vi "Change AO Gain On Fly or Not (scaled data).vi"() -> ()   [LabVIEW 2015]
doc: "I. Description:\nThis example demonstrates how to output a continuous periodic waveform using an internal sample clock.\n\nII. Instructions for Running:\n1. Select the Physical Channel to correspond to where your signal is output on the DAQ device.\n2. Enter the Minimum and Maximum Voltage Ranges\n3. Specify the Desired Frequency of the output Waveform\n4. Enter the Waveform Information. See the documentation of the Waveform Buffer Generation SubVI for information on each parameter.\n\nIII. Block Diagram Steps:\n1. Create an Analog Output Voltage channel.\n2. Call the DAQmx Timing (Use Waveform) VI which sets the sample clock rate based on the input waveform parameters, and set the sample mode to Continuous.\n3. Write the waveform to the output buffer.\n4. Call the Start VI.\n5. Loop continuously until the user presses the Stop button. Check for errors every 100 ms using the Is Task Done? VI\n6. Clear the Task\n7. Use the popup dialog box to display an error or warning if any.\n\nIV. I/O Connections Overview:\nMake sure your signal output terminal matches the Physical Channel I/O Control. For further connection information, refer to your hardware reference manual."
uses:
  <vilib>/DAQmx/create/channels.llb/DAQmx Create Channel (AO-Voltage-Basic).vi
  <vilib>/Utility/error.llb/DialogType.ctl
  <vilib>/DAQmx/configure/timing.llb/DAQmx Timing (Sample Clock).vi
  <vilib>/DAQmx/write.llb/DAQmx Write (Analog 2D DBL NChan NSamp).vi
  <resource>/objmgr/daqmx.rc
panel:
  in  "AO Idle State":bool=TRUE
  in  "Gain Setting 2":u16(ring) items=["0 dB Gain"=0, "20 dB Gain"=2, "40 dB Gain"=4]
  in  "AO Channel 2":u16(ring)=1536 items=["AO 0"=1536, "AO 1"=1540]
  in  "AO Channel":u16(ring)=1536 items=["AO 0"=1536, "AO 1"=1540]
  in  "Gain Setting":u16(ring) items=["0 dB Gain"=0, "20 dB Gain"=2, "40 dB Gain"=4]
  out "Resulting Frequency":dbl=1000.0000002037268 format="%.2f"
  in  "Cycles per Buffer":i32=5
  in  "Waveform Type":T1(ring)
  in  "Desired Frequency":dbl=1000.0 format="%.2f"
  in  "Samples per Buffer":dbl=250.0
  in  "Amplitude":dbl=10.0 format="%0.2p"
  out "Waveform Graph":dbl[](graph)=[0.0, 1.2533323356430426, 2.486898871648548, 3.6812455268467796, 4.817536741017153, 5.877852522924731, 6.845471059286887, 7.705132427757892, 8.443279255020151, 9.048270524660195, 9.510565162951536, 9.822872507286887, 9.980267284282716, 9.980267284282716, 9.822872507286887, 9.510565162951536, 9.048270524660195, 8.443279255020151, 7.705132427757892, 6.845471059286886, 5.877852522924731, 4.817536741017152, 3.681245526846779, 2.4868988716485467, 1.2533323356430417, -1.7390602846667491e-15, -1.2533323356430437, -2.4868988716485503, -3.6812455268467814, -4.817536741017156, -5.877852522924734, -6.84547105928689, -7.705132427757895, -8.443279255020155, -9.048270524660198, -9.51056516295154, -9.82287250728689, -9.98026728428272, -9.980267284282718, -9.82287250728689, -9.510565162951536, -9.048270524660198, -8.443279255020151, -7.705132427757895, -6.845471059286886, -5.877852522924733, -4.817536741017151, -3.6812455268467796, -2.4868988716485454, -1.2533323356430413, 3.432800918523604e-15, 1.253332335643045, 2.486898871648552, 3.6812455268467836, 4.8175367410171575, 5.877852522924736, 6.845471059286892, 7.705132427757898, 8.443279255020155, 9.048270524660202, 9.51056516295154, 9.822872507286894, 9.98026728428272, 9.980267284282721, 9.82287250728689, 9.51056516295154, 9.048270524660197, 8.443279255020153, 7.705132427757892, 6.845471059286887, 5.877852522924729, 4.817536741017152, 3.681245526846776, 2.486898871648546, 1.2533323356430375, -3.4618575367462157e-15, -1.2533323356430486, -2.486898871648553, -3.6812455268467863, -4.817536741017159, -5.877852522924738, -6.8454710592868935, -7.705132427757898, -8.443279255020158, -9.0482705246602, -9.510565162951544, -9.82287250728689, -9.980267284282723, -9.980267284282718, -9.822872507286894, -9.510565162951536, -9.0482705246602, -8.44327925502015, -7.705132427757895, -6.845471059286884, -5.877852522924731, -4.817536741017148, -3.6812455268467765, -2.486898871648541, -1.253332335643037, 8.040009630283507e-15, 1.2533323356430497, 2.4868988716485565, 3.681245526846788, 4.817536741017162, 5.877852522924741, 6.845471059286895, 7.705132427757902, 8.443279255020158, 9.048270524660204, 9.510565162951542, 9.822872507286894, 9.98026728428272, 9.980267284282721, 9.822872507286888, 9.51056516295154, 9.048270524660195, 8.443279255020153, 7.705132427757889, 6.845471059286886, 5.8778525229247265, 4.8175367410171495, 3.681245526846773, 2.486898871648542, 1.2533323356430341, -8.543513119185775e-15, -1.2533323356430521, -2.4868988716485583, -3.6812455268467903, -4.817536741017165, -5.8778525229247425, -6.8454710592869, -7.705132427757903, -8.443279255020164, -9.048270524660204, -9.510565162951547, -9.822872507286894, -9.980267284282725, -9.98026728428272, -9.822872507286894, -9.510565162951538, -9.048270524660198, -8.443279255020151, -7.705132427757892, -6.845471059286885, -5.877852522924727, -4.817536741017148, -3.6812455268467725, -2.4868988716485405, -1.2533323356430324, 8.901516676540489e-15, 1.253332335643055, 2.486898871648558, 3.681245526846794, 4.817536741017164, 5.877852522924746, 6.845471059286898, 7.705132427757906, 8.44327925502016, 9.048270524660207, 9.510565162951544, 9.822872507286897, 9.980267284282721, 9.980267284282723, 9.82287250728689, 9.51056516295154, 9.048270524660195, 8.443279255020151, 7.705132427757889, 6.845471059286884, 5.877852522924726, 4.817536741017146, 3.681245526846771, 2.486898871648538, 1.2533323356430321, -1.2734388196711244e-14, -1.253332335643054, -2.4868988716485623, -3.681245526846791, -4.817536741017168, -5.8778525229247425, -6.8454710592869015, -7.705132427757903, -8.443279255020164, -9.048270524660204, -9.510565162951547, -9.822872507286894, -9.980267284282725, -9.98026728428272, -9.822872507286892, -9.510565162951536, -9.048270524660197, -8.44327925502015, -7.705132427757889, -6.845471059286883, -5.877852522924725, -4.817536741017146, -3.6812455268467694, -2.4868988716485387, -1.253332335643029, 1.1011590944631777e-14, 1.2533323356430581, 2.4868988716485605, 3.6812455268467965, 4.8175367410171654, 5.877852522924749, 6.845471059286899, 7.705132427757909, 8.443279255020162, 9.04827052466021, 9.510565162951545, 9.822872507286899, 9.980267284282723, 9.980267284282725, 9.82287250728689, 9.51056516295154, 9.048270524660195, 8.443279255020151, 7.7051324277578885, 6.845471059286883, 5.877852522924724, 4.817536741017144, 3.681245526846769, 2.486898871648535, 1.253332335643029, -1.612208630485945e-14, -1.2533323356430577, -2.4868988716485663, -3.6812455268467956, -4.8175367410171726, -5.877852522924747, -6.845471059286907, -7.705132427757906, -8.443279255020169, -9.048270524660207, -9.510565162951552, -9.822872507286895, -9.980267284282728, -9.980267284282721, -9.822872507286895, -9.510565162951538, -9.048270524660198, -8.44327925502015, -7.70513242775789, -6.845471059286881, -5.877852522924724, -4.817536741017143, -3.681245526846767, -2.486898871648535, -1.2533323356430262] caption="Output Waveform"
  in  "Physical Channels":tag="PXI1Slot2/ao0:1"
  in  "Minimum Value":dbl=-10.0 format="%0.2f"
  in  "Maximum Value":dbl=10.0 format="%0.2f"
  in  "stop":bool
  # "For instructions, select Help>>Show Context Help"
  # "Channel Parameters"
  # "Timing Parameters"
  # "Waveform Information"
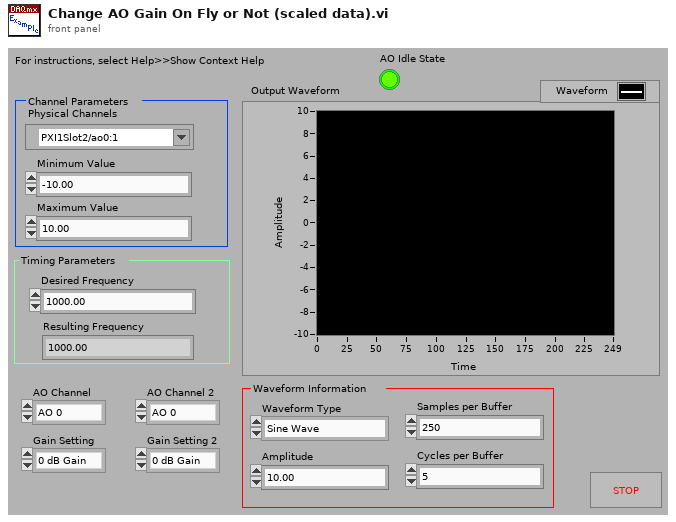
[diagram p1: front panel]
types:
  T1 = enum16{"Sine Wave", "Triangle Wave", "Square Wave", "Sawtooth Wave"}
  T2 = typedef "DialogType.ctl" = u16
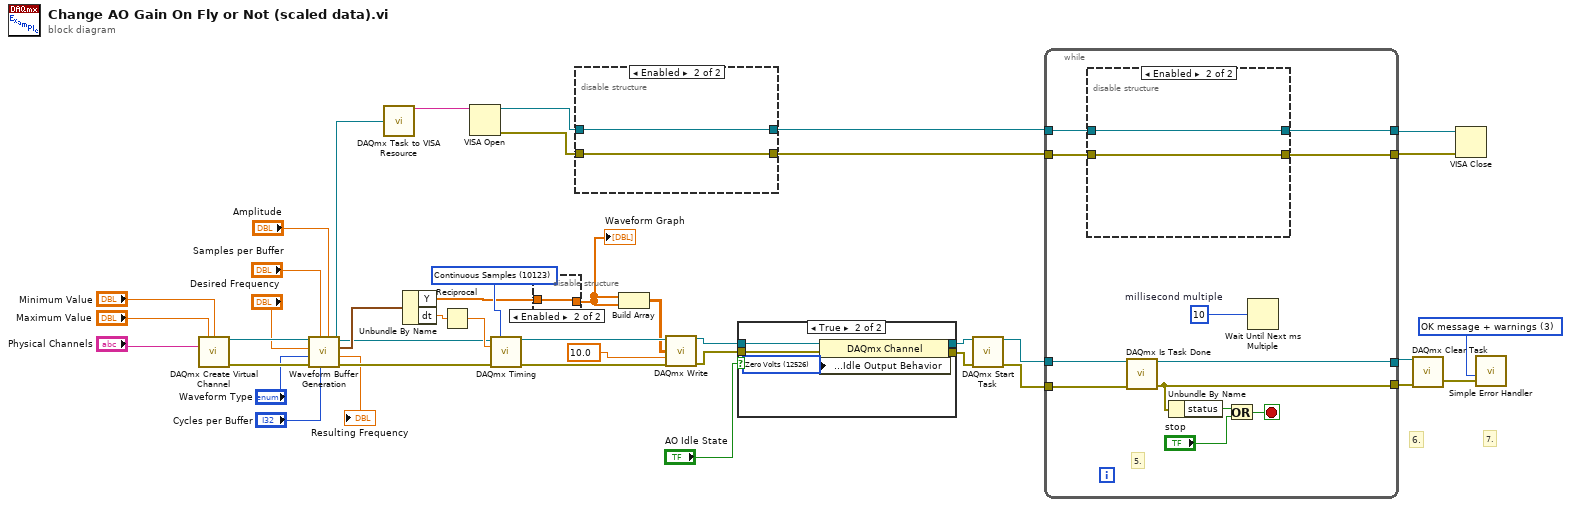
[diagram p0: block diagram]
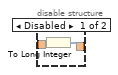
[diagram p3: hidden frame]
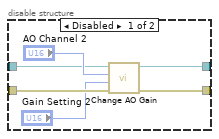
[diagram p4: hidden frame]
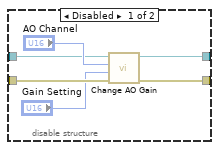
[diagram p5: hidden frame]
diagram:
  w15 = 10123 items=["Finite Samples"=10178, "Continuous Samples"=10123, "Hardware Timed Single Point"=12522] ("sample mode")
  w32 = T2 3 items=["no dialog", "OK message", "continue or stop message", "OK message + warnings", "continue/stop + warnings"] ("type of dialog (OK msg:1)")
  # "7."
  # "6."
  n1 = call-poly <vilib>:"DAQmx Create Virtual Channel.vi"("maximum value"="Maximum Value", "minimum value"="Minimum Value", "physical channels"="Physical Channels") -> ("task out"=w28:refnum<k21>, "error out"=w27:errorcluster)  [unwired: 11 in]
  n2 = call "Waveform Buffer Generation.vi"("Amplitude"="Amplitude", "Cycles per Buffer"="Cycles per Buffer", "Samples per Buffer"="Samples per Buffer", "error in (no error)"=w27, "Waveform Type"="Waveform Type", "Desired Frequency"="Desired Frequency", "task/channels in"=w28) -> ("error out"=w29:errorcluster, "Resulting Frequency"=→"Resulting Frequency":dbl, "Waveform"=w18:waveform(dbl), "task out"=w10:refnum<k21>)  [unwired: 1 out]
  n3 = call "DAQmx Task to VISA Resource.vi"("task out"=w10) -> ("VISAName"=w21:string)
  n4 = Unbundle By Name(w18) -> ("Y"=w11:dbl[], "dt"=w17:dbl)
  n5 = Reciprocal(x=w17) -> (1/x=w16:dbl)
  n6 = VISA Open(VISA resource name=w21) -> (VISA resource name=w7:refnum<visa-resource-name>, error out=w6:errorcluster)  [unwired: 4 in]
  n7 = call-poly <vilib>:"DAQmx Timing.vi"("task/channels in"=w10, "sample mode"=w15, "rate"=w16, "error in"=w29) -> ("task out"=w35:refnum<k21>, "error out"=w34:errorcluster)  [unwired: 10 in]
  n8 = disable-structure shown="Enabled" {
    disable-tunnel: [w43 w44] -> w12
    disable-tunnel: w11 -> [w42 w44]
    frame Disabled {
      n9 = To Long Integer(number=w42) -> (32bit integer=w43:i32[])
    }
    frame Enabled {
    }
  }
  "Waveform Graph" <- w12
  n10 = disable-structure shown="Enabled" {
    disable-tunnel: w6 -> [w50 w51]
    disable-tunnel: [w49 w52] -> w9
    disable-tunnel: [w48 w51] -> w8
    disable-tunnel: w7 -> [w45 w52]
    frame Disabled {
      n11 = call "Change AO Gain.vi"("error in"=w50, "Gain Setting"="Gain Setting 2", "AO Channel"="AO Channel 2", "VISA resource name 2"=w45) -> ("error out"=w48:errorcluster, "VISA resource name"=w49:refnum<visa-resource-name>)  [unwired: 4 in]
    }
    frame Enabled {
    }
  }
  n12 = Build Array(w12, w12) -> (w14:dbl[][])
  n13 = call-poly <vilib>:"DAQmx Write.vi"("task/channels in"=w35, "data"=w14, "timeout"=10.0 ("Wirite Timeout"), "error in"=w34) -> ("task out"=w4:refnum<k21>, "error out"=w3:errorcluster)  [unwired: 9 in, 1 out]
  n14 = case shown="True" "AO Idle State" {
    tunnel: w4 -> [w54 w58]
    tunnel: w3 -> [w53 w57]
    tunnel: [w54 w56] -> w2
    tunnel: [w53 w55] -> w1
    frame False {
    }
    frame True {
      w59 = 12526 items=["Zero Volts"=12526, "High Impedance"=12527, "Maintain Existing Value"=12528] ("AO.IdleOutputBehavior")
      n15 = property class="DAQmx Channel"(reference=w58, error in=w57, "Analog Output:General Properties:Output Configuration:Idle Output Behavior"=w59) -> (reference out=w56:refnum<k21>, error out=w55:errorcluster)
    }
  }
  n16 = call <vilib>:"DAQmx Start Task.vi"("task/channels in"=w2, "error in"=w1) -> ("task out"=w33:refnum<k21>, "error out"=w37:errorcluster)  [unwired: 12 in]
  n17 = while {
    tunnel: w33 -> [w71]
    tunnel: [w70] -> w31
    tunnel: w37 -> [w69]
    tunnel: [w68] -> w30
    tunnel: w9 -> [w60]
    tunnel: w8 -> [w63]
    tunnel: [w62] -> w20
    tunnel: [w61] -> w19
    stop <- w66 stop-if-true
    w67 = u32 10  # millisecond multiple
    # "5."
    n18 = disable-structure shown="Enabled" {
      disable-tunnel: w63 -> [w77 w78]
      disable-tunnel: [w76 w79] -> w62
      disable-tunnel: [w75 w78] -> w61
      disable-tunnel: w60 -> [w72 w79]
      frame Disabled {
        n19 = call "Change AO Gain.vi"("error in"=w77, "Gain Setting"="Gain Setting", "AO Channel"="AO Channel", "VISA resource name 2"=w72) -> ("error out"=w75:errorcluster, "VISA resource name"=w76:refnum<visa-resource-name>)  [unwired: 4 in]
      }
      frame Enabled {
      }
    }
    n20 = call <vilib>:"DAQmx Is Task Done.vi"("task/channels in"=w71, "error in"=w69) -> ("task out"=w70:refnum<k21>, "error out"=w68:errorcluster)  [unwired: 11 in, 1 out]
    n21 = Unbundle By Name(w68) -> ("status"=w65:bool)
    n22 = Or(x=w65, y="stop") -> (x .or. y?=w66:bool)
    n23 = Wait Until Next ms Multiple(millisecond multiple=w67) -> ()  [unwired: 1 out]
  }
  n24 = call <vilib>:"DAQmx Clear Task.vi"("task in"=w31, "error in"=w30) -> ("error out"=w41:errorcluster)  [unwired: 13 in]
  n25 = VISA Close(VISA resource name=w20, error in (no error)=w19) -> ()  [unwired: 1 out]
  n26 = call <vilib>:"Simple Error Handler.vi"("type of dialog (OK msg:1)"=w32, "error in (no error)"=w41) -> ()  [unwired: 3 in, 5 out]
